vi "Modbus TCP Close.vi"(8 "error in (no error)":errorcluster, 11 "MB session in":refnum<class "MB_Master.lvclass">) -> (0 "error out":errorcluster)   [LabVIEW 2024, in "Bronkhorst Flexi-Flow ModbusTCP API.lvlib"]
uses:
  Bronkhorst Flexi-Flow ModbusTCP API.lvlib
  <vilib>/Plasmionique/MB Master/MB_Master/MB_Master.lvclass
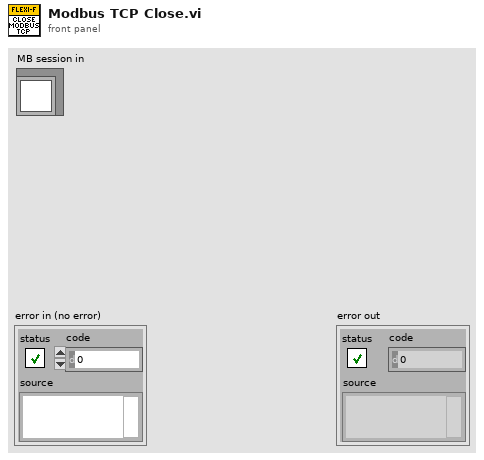
[diagram p1: front panel]
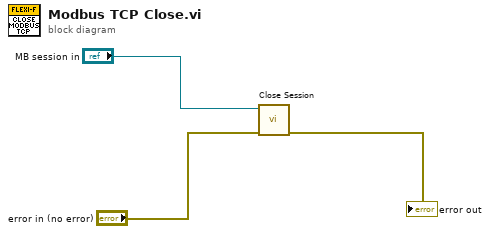
[diagram p0: block diagram]
diagram:
  n1 = call-dynamic "Close Session.vi"("error in (no error)"="error in (no error)", "MB session in"="MB session in") -> ("error out"=→"error out":errorcluster)  [unwired: 9 in]
